vi "Test Case, Charger Is Ready.vi"() -> ()   [LabVIEW 2010]
uses:
  Charger/Charger_Status Control.ctl
  Drivers/Charger Test Set/Charger_Input Control.ctl
panel:
  out "Charge Status":T1={"MICS ID"=4417, "VBAT"=nan, "ChargingState"="", "VBAT Slide"=3.5, "Status"="", "TemperatureLevel"=nan, "IPG_ReceivedLevel"=nan, "VBAT Target"=nan, "Charger Setpoint"=nan, "Index"=0, "Ready"=TRUE, "Charger Inputs"={"address"="COM17", "position"=0, "setpoint"=7500.0}, "MICS Inputs"={"address"="", "chan"=2, "ID"=0}} {"MICS Inputs"."ID" format="%04x"; "MICS Inputs"."chan" min=1 max=10 step=1; "Charger Inputs"."setpoint" min=0.0 max=20000.0 step=100.0; "Charger Inputs"."position" min=0 max=5 step=1; "MICS ID" format="%04x"; "VBAT Target" format="%.2f"; "VBAT Slide" scale=3.5..4.0 scale format="%.2f"; "VBAT" format="%.2f"}
  out "ready":bool
  in  "stop":bool
  out "error out":errorcluster
  in  "error in":errorcluster
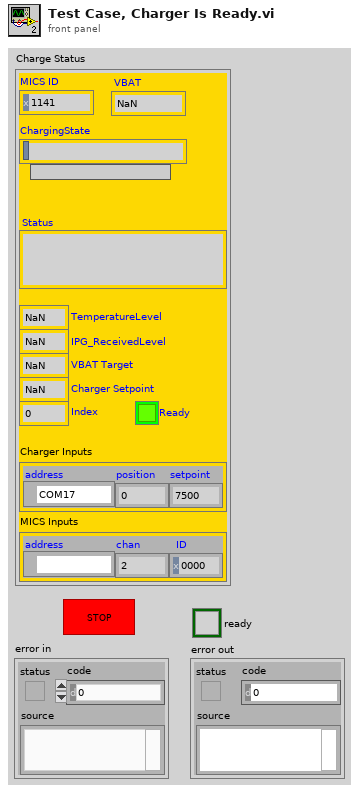
[diagram p1: front panel]
types:
  T1 = typedef "Charger_Status Control.ctl" = cluster{"MICS ID":u32, "VBAT":dbl, "ChargingState":string, "VBAT Slide":dbl, "Status":string, "TemperatureLevel":dbl, "IPG_ReceivedLevel":dbl, "VBAT Target":dbl, "Charger Setpoint":dbl, "Index":i32, "Ready":bool, "Charger Inputs":T2, "MICS Inputs":cluster{"address":refnum<visa-resource-name>, "chan":u16, "ID":u32}}
  T2 = typedef "Charger_Input Control.ctl" = cluster{"address":refnum<visa-resource-name>, "position":i32, "setpoint":dbl}
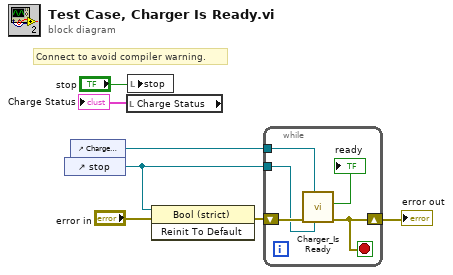
[diagram p0: block diagram]
diagram:
  # "Connect to avoid compiler warning."
  n1 = control-ref of="stop"() -> (w6:refnum<vi>)
  n2 = control-ref of="Charge Status"() -> (w1:refnum<vi>)
  n3 = local read "Charge Status"() -> (→"Charge Status":T1)
  n4 = local write "stop"("stop") -> ()
  n5 = invoke class="Bool (strict)" method="Reinit To Default"(reference=w6, error in="error in") -> (error out=w4:errorcluster)  [unwired: 1 in, 2 out]
  n6 = while {
    tunnel: w6 -> [w10]
    shift-right: [w11] -> w7
    shift-left: w4 -> [w12]
    tunnel: w1 -> [w9]
    stop <- w11 stop-if-true
    n7 = call "Charger_Is Ready.vi"("Stop Refnum"=w10, "Status Refnum"=w9, "error in"=w12) -> ("error out"=w11:errorcluster, "ready"=→"ready":bool)  [unwired: 7 in]
  }
  "error out" <- w7
